vi "TestSecondsCheck.vi"() -> ()   [LabVIEW 2012]
uses:
  <vilib>/addons/database/Connection.llb/DB Tools Open Connec (Path).vi
  <vilib>/addons/database/Connection.llb/Conn Execute.vi
  <vilib>/addons/database/Recordset.llb/Rec Fetch Recordset Data (R).vi
  <vilib>/addons/database/Recordset.llb/Rec Destroy - Connection.vi
  <vilib>/addons/database/Recordset.llb/Rec Fetch Integer Data (R).vi
  <vilib>/addons/database/_DB Variant To Data/Database Variant To Data.xnode
  <vilib>/addons/database/NI_Database_API.lvlib
  <vilib>/Utility/SMTP/NI_SMTPEmail.lvlib
panel:
  out "spreadsheet string":string
  out "array":string[][](array[string])
  out "appended array":string[](array[string])
  out "concatenated string":string
  out "error out":errorcluster
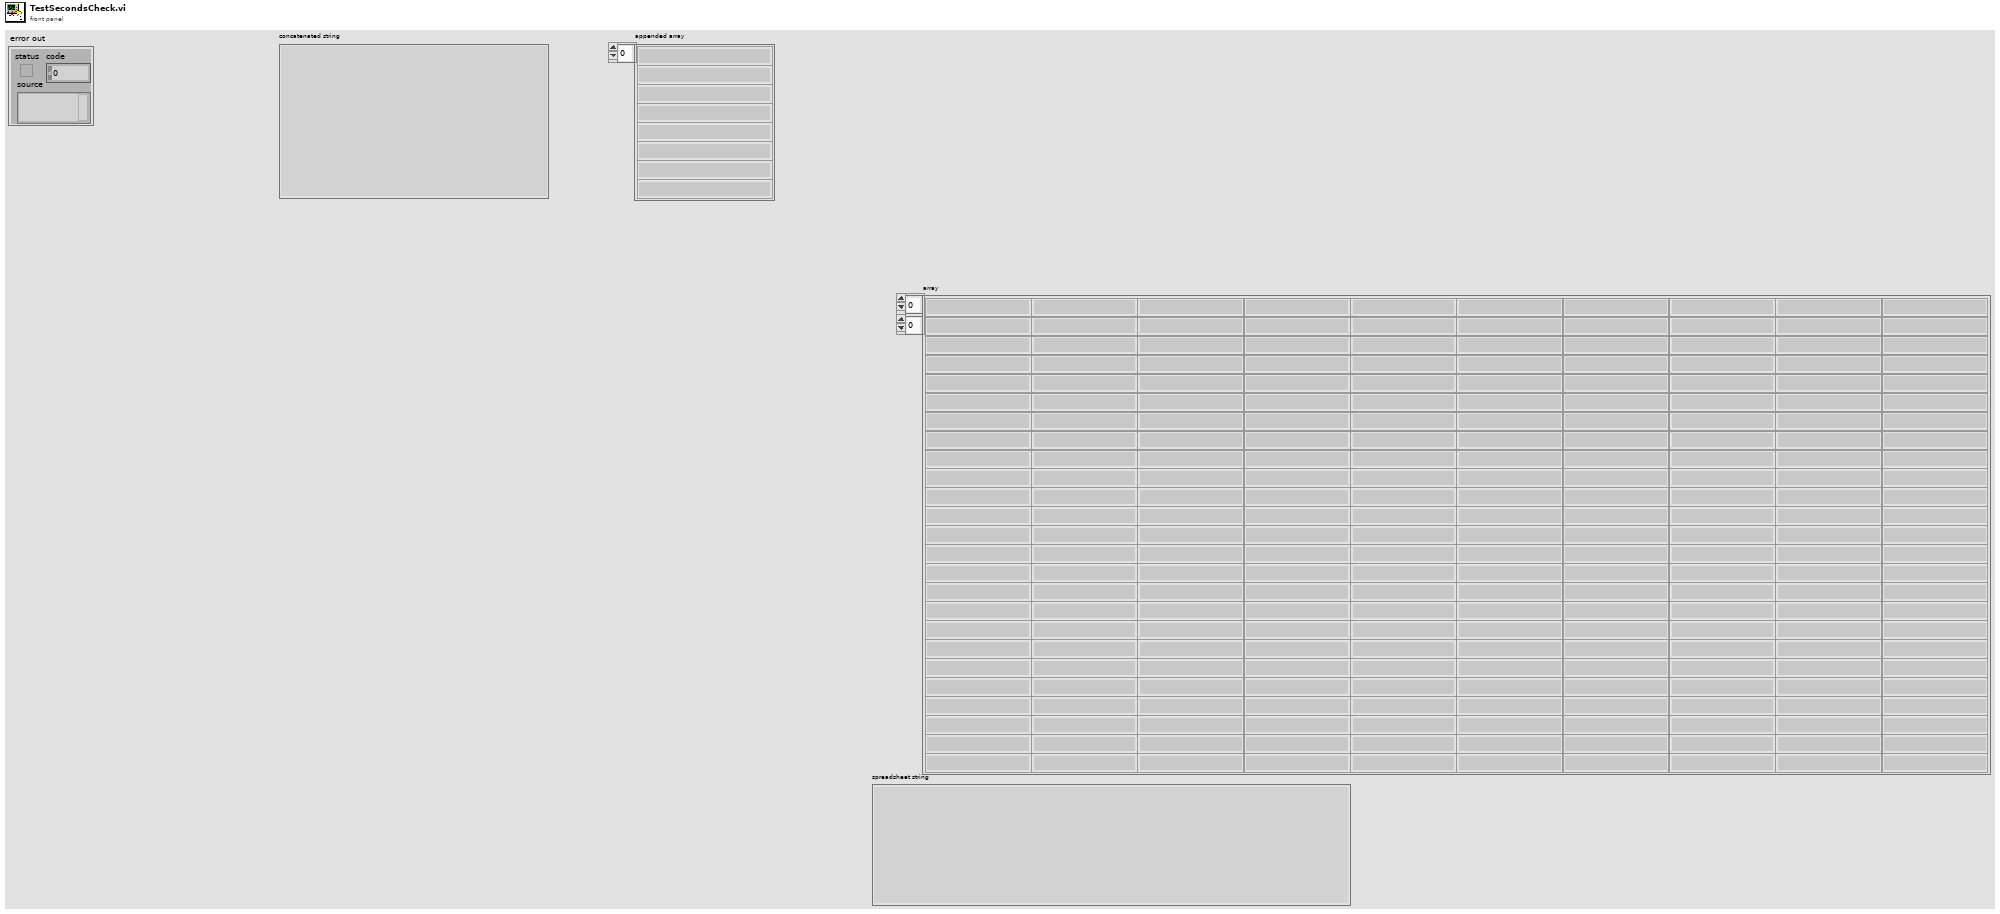
[diagram p1: front panel]
types:
  T1 = typedef "NI_Database_API.lvlib/Conn ObjectReference.ctl" = refnum<k1>
  T2 = typedef "NI_Database_API.lvlib/Rec ObjectReference.ctl" = refnum<k1>
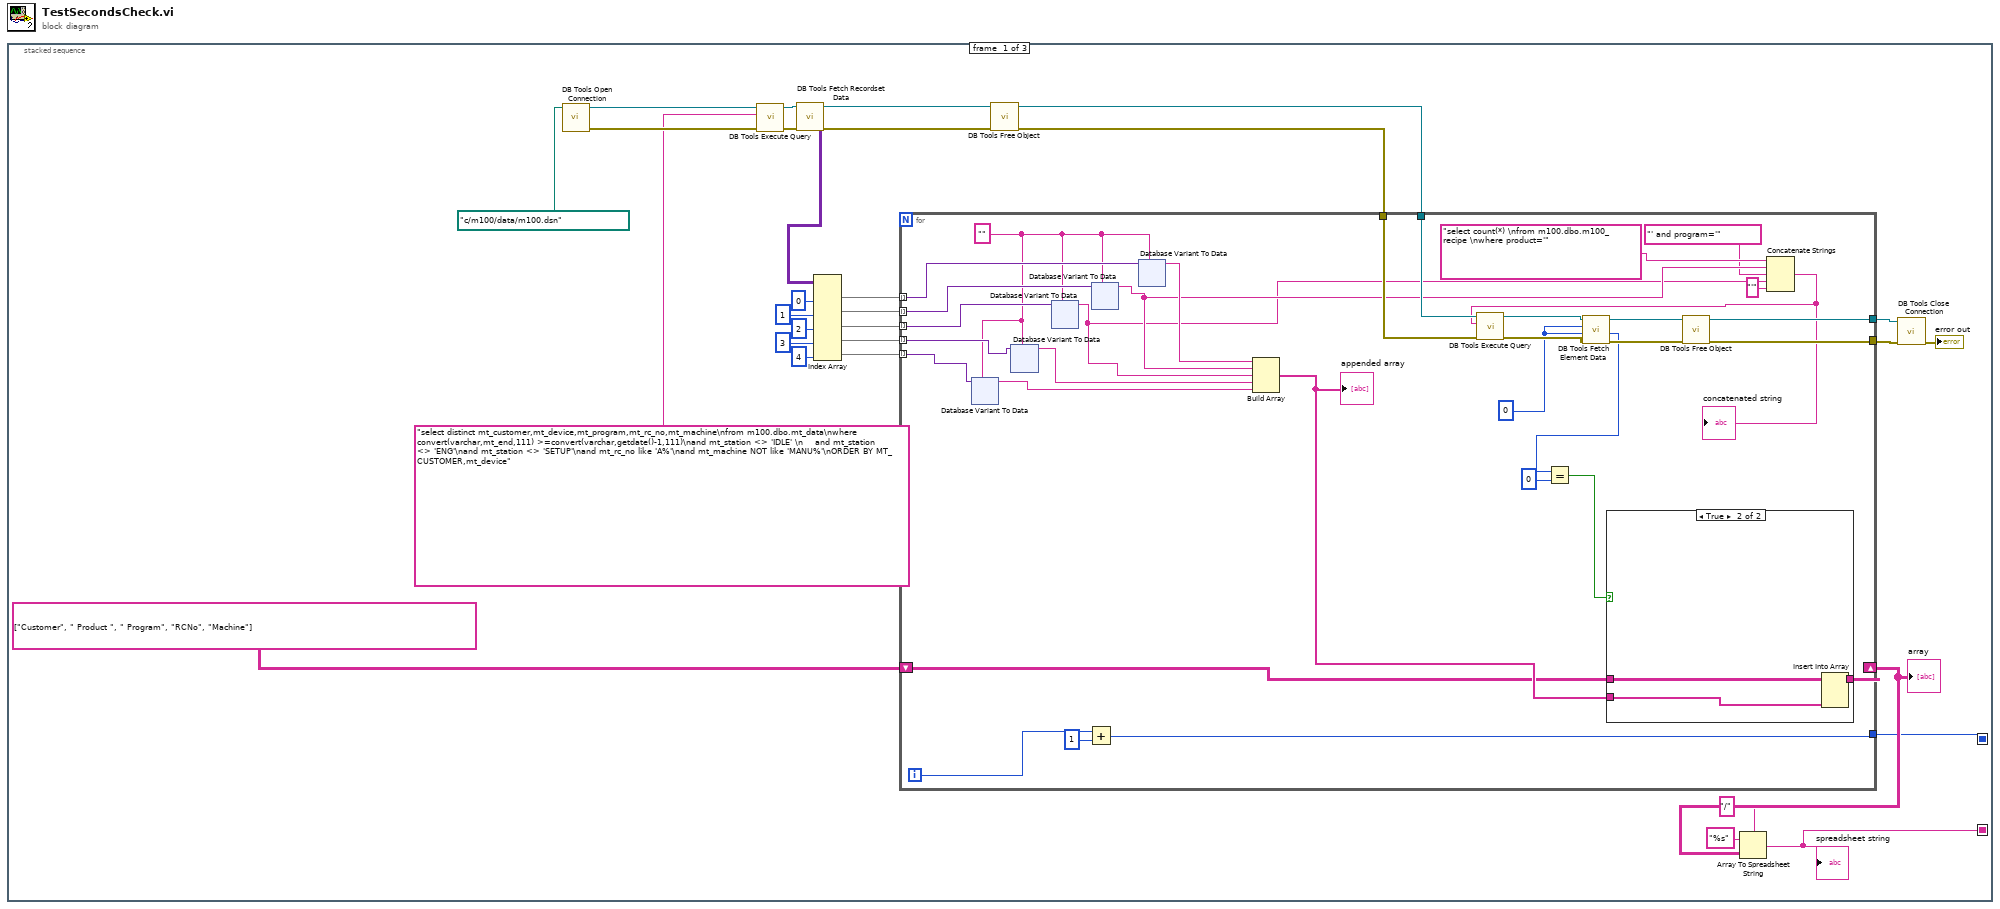
[diagram p0: block diagram]
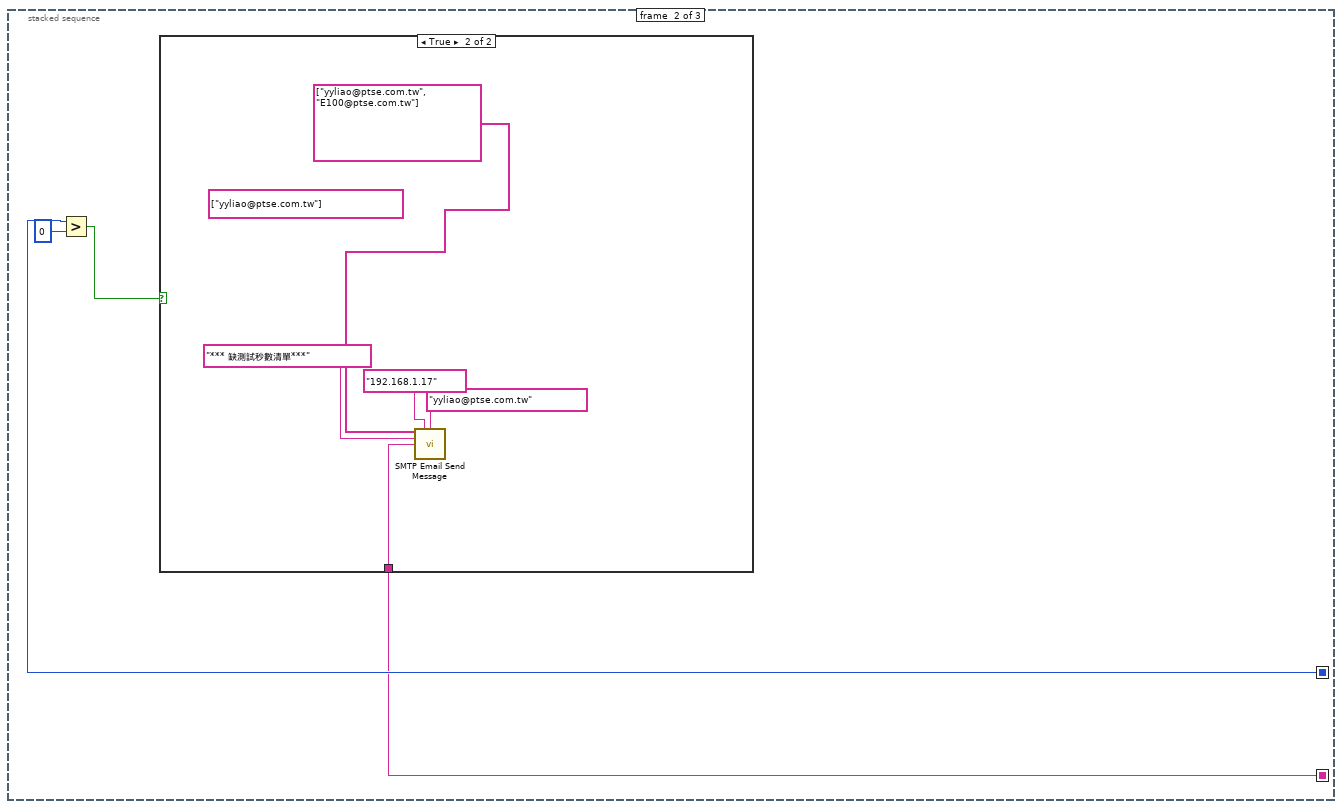
[diagram p3: hidden frame]
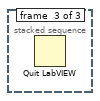
[diagram p5: hidden frame]
diagram:
  n1 = stacked-sequence {
    seq-local: [w6 _ _] -> [_ w230 _]
    seq-local: [w5 _ _] -> [_ w229 _]
    frame #0 {
      n2 = call-poly <vilib>:"DB Tools Open Connection.vi"("connection information"=path "c:/m100/data/m100.dsn") -> ("error out"=w27:errorcluster, "connection reference"=w30:T1)  [unwired: 7 in]
      n3 = call-poly <vilib>:"DB Tools Execute Query.vi"("error in (no error)"=w27, "SQL query"="select distinct mt_customer,mt_device,mt_program,mt_rc_no,mt_machine\nfrom m100.dbo.mt_data\nwhere convert(varchar,mt_end,111) >=convert(varchar,getdate()-1,111)\nand mt_station <> 'IDLE' \n    and mt_station <> 'ENG'\nand mt_station <> 'SETUP'\nand mt_rc_no like 'A%'\nand mt_machine NOT like 'MANU%'\nORDER BY MT_CUSTOMER,mt_device", "connection reference"=w30) -> ("error out"=w26:errorcluster, "recordset reference"=w29:T2)  [unwired: 5 in]
      n4 = call-poly <vilib>:"DB Tools Fetch Recordset Data.vi"("error in (no error)"=w26, "recordset reference"=w29) -> ("error out"=w25:errorcluster, "recordset data"=w21:variant[][], "recordset reference out"=w28:T2)  [unwired: 3 in]
      n5 = Index Array(array=w21, index (col) #1=0 ("disabled index (col)"), index (col) #2=1 ("index (col)"), index (col) #3=2 ("index (col)"), index (col) #4=3 ("index (col)"), index (col) #5=4 ("index (col)")) -> (element #1=w15:variant[], element #2=w16:variant[], element #3=w17:variant[], element #4=w2:variant[], element #5=w1:variant[])  [unwired: 5 in]
      n6 = call-poly <vilib>:"DB Tools Free Object.vi"("error in (no error)"=w25, "recordset reference"=w28) -> ("error out"=w13:errorcluster, "connection reference"=w14:T1)  [unwired: 8 in]
      n7 = for {
        tunnel: w17 -> [w63] mode=indexing
        tunnel: w16 -> [w62] mode=indexing
        tunnel: w15 -> [w61] mode=indexing
        tunnel: w14 -> [w59]
        tunnel: w13 -> [w58]
        tunnel: [w53] -> w12
        tunnel: [w52] -> w11
        shift-right: [w41] -> w8
        shift-left: string[][] [["Customer", " Product ", " Program", "RCNo", "Machine"]] ("array") -> [w40]
        tunnel: [w36] -> w6
        tunnel: w2 -> [w35] mode=indexing
        tunnel: w1 -> [w34] mode=indexing
        i -> [w37]
        w46 = 0
        w33 = ""
        n8 = xnode "Database Variant To Data"("database variant"=w34, "type"=w33) -> ("data"=w31:string)  [unwired: 1 in, 1 out]
        n9 = xnode "Database Variant To Data"("database variant"=w35, "type"=w33) -> ("data"=w32:string)  [unwired: 1 in, 1 out]
        n10 = xnode "Database Variant To Data"("database variant"=w63, "type"=w33) -> ("data"=w39:string)  [unwired: 1 in, 1 out]
        n11 = Add(x=w37, y=1) -> (x+y=w36:i32)
        n12 = xnode "Database Variant To Data"("database variant"=w62, "type"=w33) -> ("data"=w50:string)  [unwired: 1 in, 1 out]
        n13 = xnode "Database Variant To Data"("database variant"=w61, "type"=w33) -> ("data"=w60:string)  [unwired: 1 in, 1 out]
        n14 = Build Array(w60, w50, w39, w32, w31) -> (w42:string[])
        "appended array" <- w42
        n15 = Concatenate Strings("select count(*) \nfrom m100.dbo.m100_recipe \nwhere product='" ("SQL query"), w50, "' and program='" ("string"), w39, "'" ("string")) -> (w48:string)
        "concatenated string" <- w48
        n16 = call-poly <vilib>:"DB Tools Execute Query.vi"("error in (no error)"=w58, "SQL query"=w48, "connection reference"=w59) -> ("error out"=w56:errorcluster, "recordset reference"=w57:T2)  [unwired: 5 in]
        n17 = call-poly <vilib>:"DB Tools Fetch Element Data.vi"("error in (no error)"=w56, "type"=w46, "column index"=w46, "recordset reference"=w57) -> ("error out"=w54:errorcluster, "data"=w45:i32, "recordset reference out"=w55:T2)  [unwired: 3 in]
        n18 = Equal?(x=w45, y=0) -> (x = y?=w43:bool)
        n19 = case shown="True" w43 {
          tunnel: [w128 w131] -> w41
          tunnel: w42 -> [_ w130]
          tunnel: w40 -> [w128 w129]
          frame False {
          }
          frame True {
            n20 = Insert Into Array(array=w129, new element=w130) -> (w131:string[][])  [unwired: 2 in]
          }
        }
        n21 = call-poly <vilib>:"DB Tools Free Object.vi"("error in (no error)"=w54, "recordset reference"=w55) -> ("error out"=w52:errorcluster, "connection reference"=w53:T1)  [unwired: 8 in]
      }
      "array" <- w8
      n22 = Array To Spreadsheet String(delimiter (Tab)="/", array=w8, 3:"%s" ("format string")) -> (spreadsheet string=w5:string)
      "spreadsheet string" <- w5
      n23 = call <vilib>:"DB Tools Close Connection.vi"("error in (no error)"=w11, "connection reference"=w12) -> ("error out"=→"error out":errorcluster)  [unwired: 5 in]
    }
    frame #1 {
      n24 = Greater?(x=w230, y=0) -> (0:w228:bool)
      n25 = case shown="True" w228 {
        tunnel: w229 -> [_ w233]
        frame False {
        }
        frame True {
          (unwired) string[] ["yyliao@ptse.com.tw"] ("recipients")
          n26 = call <vilib>:"SMTP Email Send Message.vi"("recipients"=string[] ["yyliao@ptse.com.tw", "E100@ptse.com.tw"], "mail server"="192.168.1.17", "return address"="yyliao@ptse.com.tw", "subject ([No Subject])"="*** 缺測試秒數清單***", "message"=w233) -> ()  [unwired: 9 in, 2 out]
        }
      }
    }
    frame #2 {
      n27 = Quit LabVIEW() -> ()  [unwired: 1 in]
    }
  }
